vi "Tolleranze croci.vi"() -> (2 "cancelled?":bool=TRUE)   [LabVIEW 2019]
uses:
  <vilib>/Utility/file.llb/Write Delimited Spreadsheet (string).vi
  <vilib>/Utility/file.llb/Read Delimited Spreadsheet (string).vi
panel:
  in  "Cancel Button":bool
  in  "OK Button":bool
  in  "Tolleranze croci":T1 {"EtaP[%]" format="%#_g %"; "Ptot[%]" format="%#_g %"; "Htot[%]" format="%#_g %"; "Q[%]" format="%#_g %"}
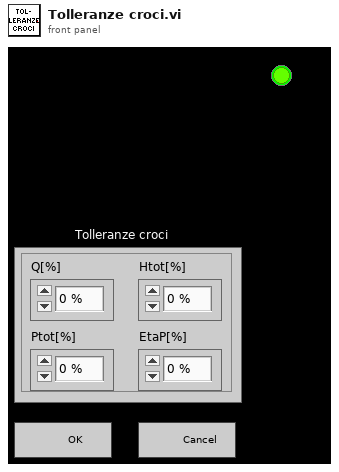
[diagram p1: front panel]
types:
  T1 = cluster{"Q[%]":dbl, "Htot[%]":dbl, "Ptot[%]":dbl, "EtaP[%]":dbl}
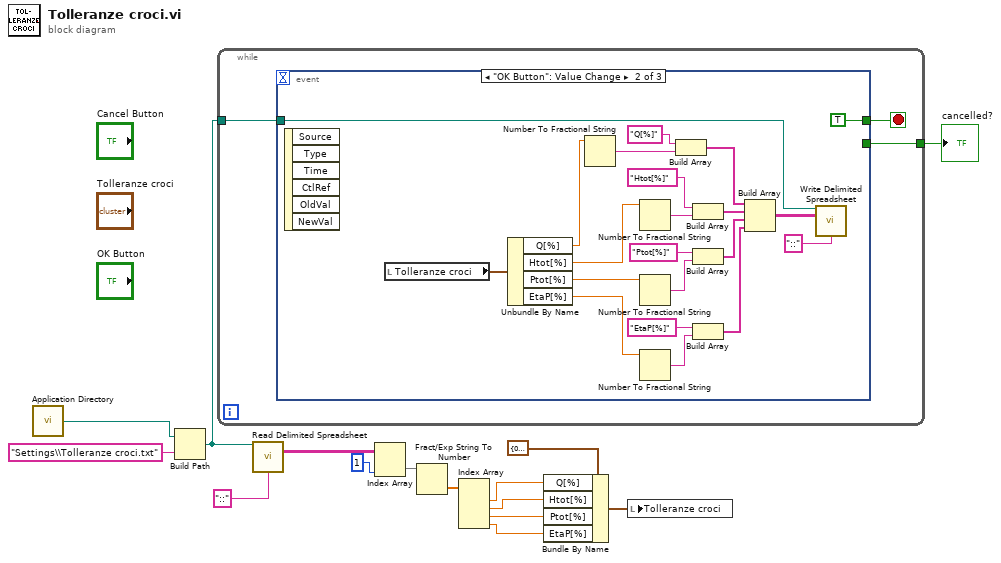
[diagram p0: block diagram]
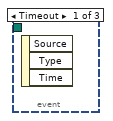
[diagram p2: hidden frame]
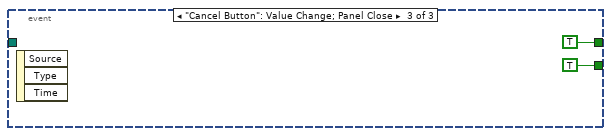
[diagram p3: hidden frame]
diagram:
  n1 = call <vilib>:"Application Directory.vi"() -> ("Application Directory"=w15:path)
  n2 = Build Path(base path=w15, name or relative path="Settings\\Tolleranze croci.txt") -> (appended path=w2:path)
  n3 = while {
    tunnel: w2 -> [w17]
    tunnel: [w16] -> w1
    stop <- w18 stop-if-true
    n4 = event shown="[1] \"OK Button\": Value Change" {
      selector: _ -> [_ _ _]
      dyn-events: _ -> [_ _ _]
      timeout: _ -> [_ _ _]
      tunnel: [_ TRUE TRUE] -> w18
      tunnel: w17 -> [_ w39 _]
      tunnel: [_ _ TRUE] -> w16
      event Timeout {
        n5 = event-data() -> ()  [unwired: 1 in, 3 out]
      }
      event "OK Button": Value Change {
        n6 = event-data() -> ()  [unwired: 1 in, 6 out]
        n7 = local read "Tolleranze croci"() -> (w22:T1)
        n8 = Unbundle By Name(w22) -> ("Q[%]"=w23:dbl, "Htot[%]"=w24:dbl, "Ptot[%]"=w25:dbl, "EtaP[%]"=w26:dbl)
        n9 = Number To Fractional String(number=w23) -> (F-format string=w27:string)  [unwired: 3 in]
        n10 = Number To Fractional String(number=w24) -> (F-format string=w32:string)  [unwired: 3 in]
        n11 = Number To Fractional String(number=w25) -> (F-format string=w33:string)  [unwired: 3 in]
        n12 = Number To Fractional String(number=w26) -> (F-format string=w34:string)  [unwired: 3 in]
        n13 = Build Array("Q[%]" ("element"), w27) -> (w35:string[])
        n14 = Build Array("Htot[%]" ("element"), w32) -> (w36:string[])
        n15 = Build Array("Ptot[%]" ("element"), w33) -> (w37:string[])
        n16 = Build Array("EtaP[%]" ("element"), w34) -> (w38:string[])
        n17 = Build Array(w35, w36, w37, w38) -> (w21:string[][])
        n18 = call-poly <vilib>:"Write Delimited Spreadsheet.vi"("file path (dialog if empty)"=w39, "2D data"=w21, "delimiter (\\t)"="::" ("delimiter (\\t)")) -> ()  [unwired: 11 in, 2 out]
      }
      event "Cancel Button": Value Change; Panel Close {
        n19 = event-data() -> ()  [unwired: 1 in, 3 out]
      }
    }
  }
  "cancelled?" <- w1
  n20 = call-poly <vilib>:"Read Delimited Spreadsheet.vi"("file path (dialog if empty)"=w2, "delimiter (\\t)"="::" ("delimiter (\\t)")) -> ("all rows"=w12:string[][])  [unwired: 8 in, 5 out]
  n21 = Index Array(array=w12, index (col)=1 ("disabled index (col)")) -> (element=w10:string[])  [unwired: 1 in]
  n22 = Fract/Exp String To Number(string=w10) -> (number=w9:dbl[])  [unwired: 3 in, 1 out]
  n23 = Index Array(array=w9) -> (element #1=w7:dbl, element #2=w6:dbl, element #3=w5:dbl, element #4=w4:dbl)  [unwired: 4 in]
  n24 = Bundle By Name(cluster=T1 {"Q[%]"=0.0, "Htot[%]"=0.0, "Ptot[%]"=0.0, "EtaP[%]"=0.0} ("Tolleranze croci"), "Q[%]"=w7, "Htot[%]"=w6, "Ptot[%]"=w5, "EtaP[%]"=w4) -> (w3:T1)
  n25 = local write "Tolleranze croci"(w3) -> ()
